vi "Forebrain 1.vi"() -> ()   [LabVIEW 2011]
uses:
  Where.ctl
  Behaviour.ctl
panel:
  in  "Current State":i32
  out "WhereAmI":T1
  in  "stop":bool
  in  "Tab Control":enum32{"Mission Planning", "Auto Mode"}(tab)
  out "Mission Definition":T2[](array[typedef])
  in  "Remove":bool
  in  "Add":bool
  in  "Behaviour":T2
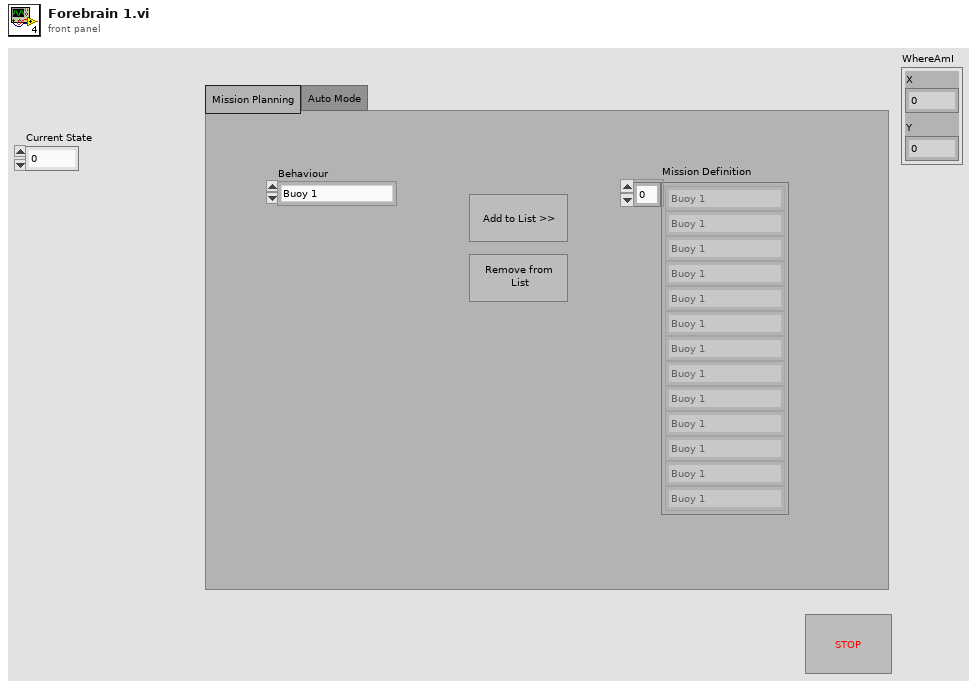
[diagram p1: front panel]
types:
  T1 = typedef "Where.ctl" = cluster{"X":dbl, "Y":dbl}
  T2 = typedef "Behaviour.ctl" = enum16{"Buoy 1", "Buoy 2", "Whale Search"}
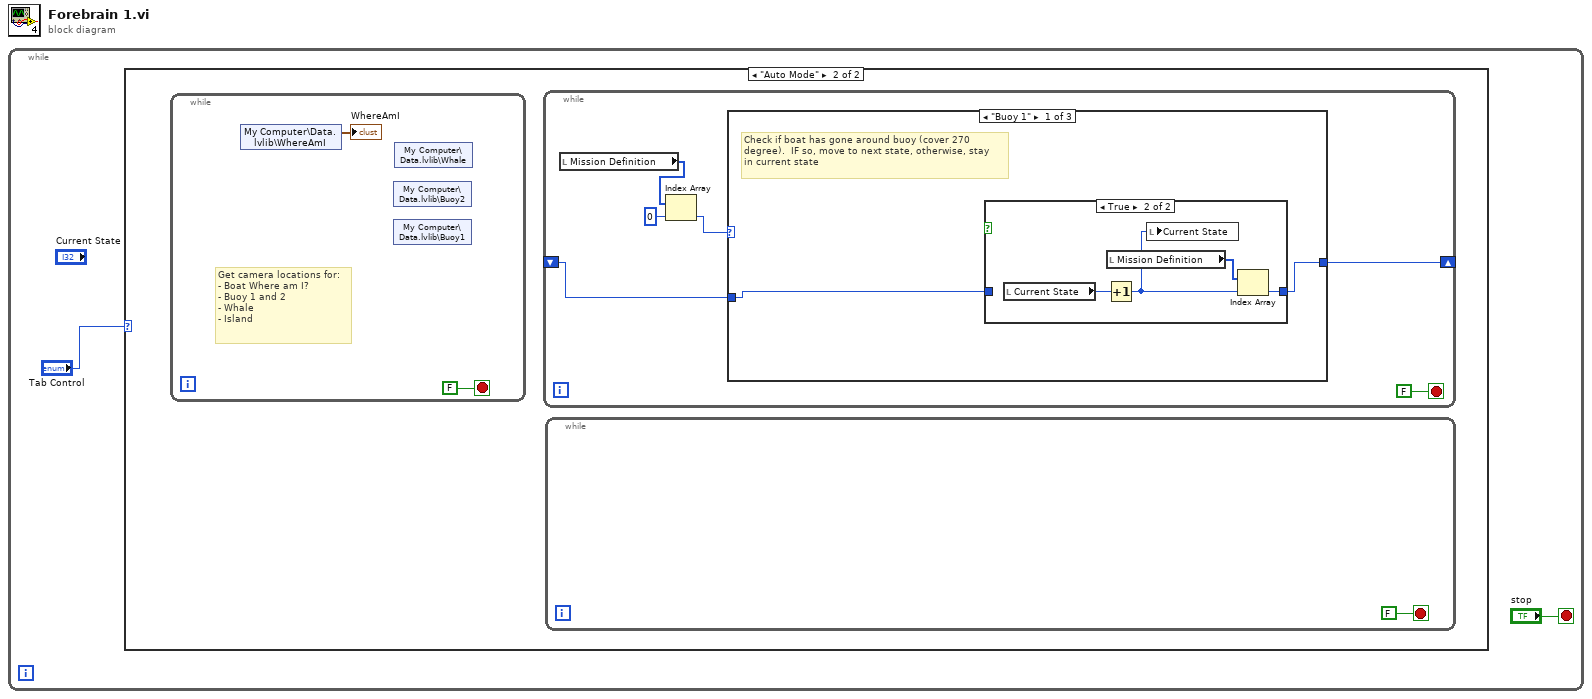
[diagram p0: block diagram]
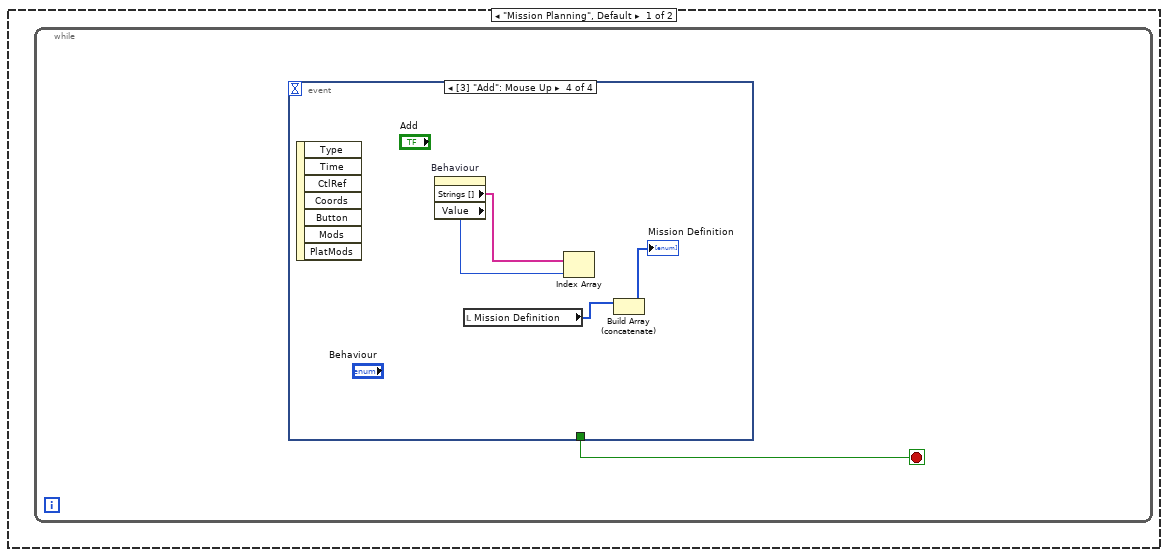
[diagram p2: hidden frame]
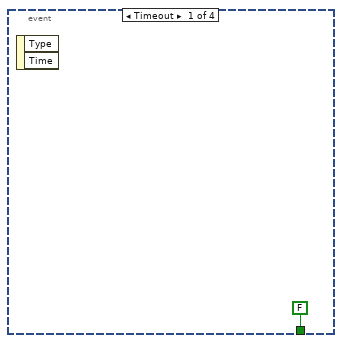
[diagram p3: hidden frame]
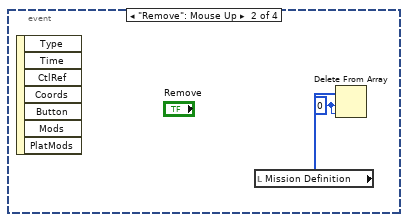
[diagram p4: hidden frame]
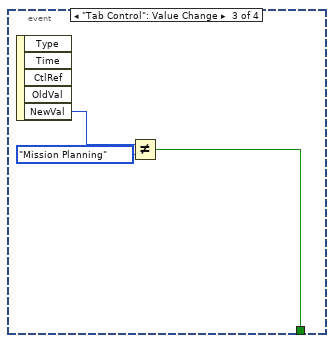
[diagram p5: hidden frame]
diagram:
  n1 = while {
    stop <- "stop" stop-if-true
    n2 = case shown="\"Auto Mode\"" "Tab Control" {
      frame "Mission Planning", Default {
        n3 = while {
          stop <- w3 stop-if-true
          n4 = event shown="[3] \"Add\": Mouse Up" {
            selector: _ -> [_ _ _ _]
            dyn-events: _ -> [_ _ _ _]
            timeout: _ -> [_ _ _ _]
            tunnel: [FALSE _ w7 _] -> w3
            event Timeout {
              n5 = event-data() -> ()  [unwired: 1 in, 2 out]
            }
            event "Remove": Mouse Up {
              w5 = 0 ("length")
              n6 = event-data() -> ()  [unwired: 1 in, 7 out]
              n7 = local read "Mission Definition"() -> (w6:T2[])
              n8 = Delete From Array(array=w6, length=w5, index=w5) -> ()  [unwired: 2 out]
            }
            event "Tab Control": Value Change {
              n9 = event-data() -> ("NewVal"=w9:enum32{"Mission Planning", "Auto Mode"})  [unwired: 1 in, 4 out]
              n10 = Not Equal?(x=w9, y=enum32{"Mission Planning", "Auto Mode"}."Mission Planning") -> (x != y?=w7:bool)
            }
            event "Add": Mouse Up {
              n11 = event-data() -> ()  [unwired: 1 in, 7 out]
              n12 = property on="Behaviour" class="Enum (strict)"() -> ("Strings []"=w13:string[], "Value"=w12:enum16{"Buoy 1", "Buoy 2", "Whale Search"})  [unwired: 2 in, 2 out]
              n13 = local read "Mission Definition"() -> (w11:T2[])
              n14 = Index Array(array=w13, index=w12) -> ()  [unwired: 1 out]
              n15 = Build Array (concatenate)(w11) -> (→"Mission Definition":T2[])  [unwired: 1 in]
            }
          }
        }
      }
      frame "Auto Mode" {
        n16 = while {
          stop <- FALSE stop-if-true
          # "Get camera locations for:\n- Boat Where am I?\n- Buoy 1 and 2\n- Whale\n- Island"
          n17 = shared-variable "My Computer\\Data.lvlib\\WhereAmI"() -> (→"WhereAmI":T1)  [unwired: 1 in, 1 out]
          n18 = shared-variable "My Computer\\Data.lvlib\\Buoy2"() -> ()  [unwired: 1 in, 2 out]
          n19 = shared-variable "My Computer\\Data.lvlib\\Buoy1"() -> ()  [unwired: 1 in, 2 out]
          n20 = shared-variable "My Computer\\Data.lvlib\\Whale"() -> ()  [unwired: 1 in, 2 out]
        }
        n21 = while {
          shift-right: [w15] -> _
          shift-left: _ -> [w16]
          stop <- FALSE stop-if-true
          n22 = local read "Mission Definition"() -> (w19:T2[])
          n23 = Index Array(array=w19, index=0) -> (element=w17:T2)
          n24 = case shown="\"Buoy 1\"" w17 {
            tunnel: w16 -> [w22 w29 w31]
            tunnel: [w21 w28 w32] -> w15
            frame "Buoy 1" {
              # "Check if boat has gone around buoy (cover 270\ndegree).  IF so, move to next state, otherwise, stay \nin current state"
              n25 = case shown="True" {
                selector: _ -> [_ _]
                tunnel: [w23 w27] -> w21
                tunnel: w22 -> [w23 _]
                frame False {
                }
                frame True {
                  n26 = local read "Current State"() -> (w26:i32)
                  n27 = Increment(x=w26) -> (x+1=w24:i32)
                  n28 = local read "Mission Definition"() -> (w25:T2[])
                  n29 = local write "Current State"(w24) -> ()
                  n30 = Index Array(array=w25, index=w24) -> (element=w27:T2)
                }
              }
            }
            frame "Buoy 2" {
              n31 = case shown="True" {
                selector: _ -> [_ _]
                tunnel: w29 -> [w30 _]
                tunnel: [w30 _] -> w28
                frame False {
                }
                frame True {
                }
              }
            }
            frame "Whale Search" {
              n32 = case shown="True" {
                selector: _ -> [_ _]
                tunnel: [_ w33] -> w32
                tunnel: w31 -> [_ w33]
                frame False {
                }
                frame True {
                }
              }
            }
          }
        }
        n33 = while {
          stop <- FALSE stop-if-true
        }
      }
    }
  }
